vi "In_S1F2.vi"(8 "error in (no error)":errorcluster, 11 "S1 Message Class in":refnum<class "S1 Message Class.lvclass">) -> (0 "error out":errorcluster, 1 "OK?":bool, 2 "S1F2":T1, 3 "S1 Message Class out":refnum<class "S1 Message Class.lvclass">)   [LabVIEW 2020, in "SECS Communication.lvlib" / "S1 Message Class.lvclass"]
uses:
  S1 Message Class.lvclass
  D:/Dropbox/SECS/SECS_GEM v1.0.6/Com/SECS Communication/SECS-II Class/SECS-II Class.lvclass
  S1F2.ctl
  SECS-II Class/SECS-II Class.lvclass/SECS-II Class.ctl
  SECS-II Class/Variant To Data_ASCII.vi
  SECS-II Class/SECS-II Class.lvclass
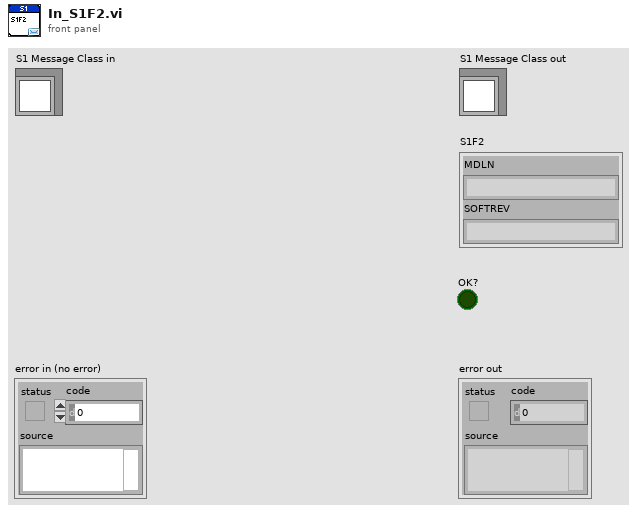
[diagram p1: front panel]
types:
  T1 = typedef "SECS Communication.lvlib/S1 Message Class.lvclass/S1F2.ctl" = cluster{"MDLN":string, "SOFTREV":string}
  T2 = typedef "SECS Communication.lvlib/SECS-II Class.lvclass/Message Data.ctl" = cluster{"Index":i32, "Data Item Format":T3, "Format Code":T4, "Parent Index":i32, "Child Index":i32[], "Data":variant}
  T3 = typedef "SECS Communication.lvlib/SECS-II Class.lvclass/Data Item Format.ctl" = enum16{"Data Type", "Value"}
  T4 = typedef "SECS Communication.lvlib/SECS-II Class.lvclass/Format Code.ctl" = enum16{"L", "A", "B", "Boolean", "J", "I1", "I2", "I4", "I8", "U1", "U2", "U4", "U8", "F4", "F8", "Char"}
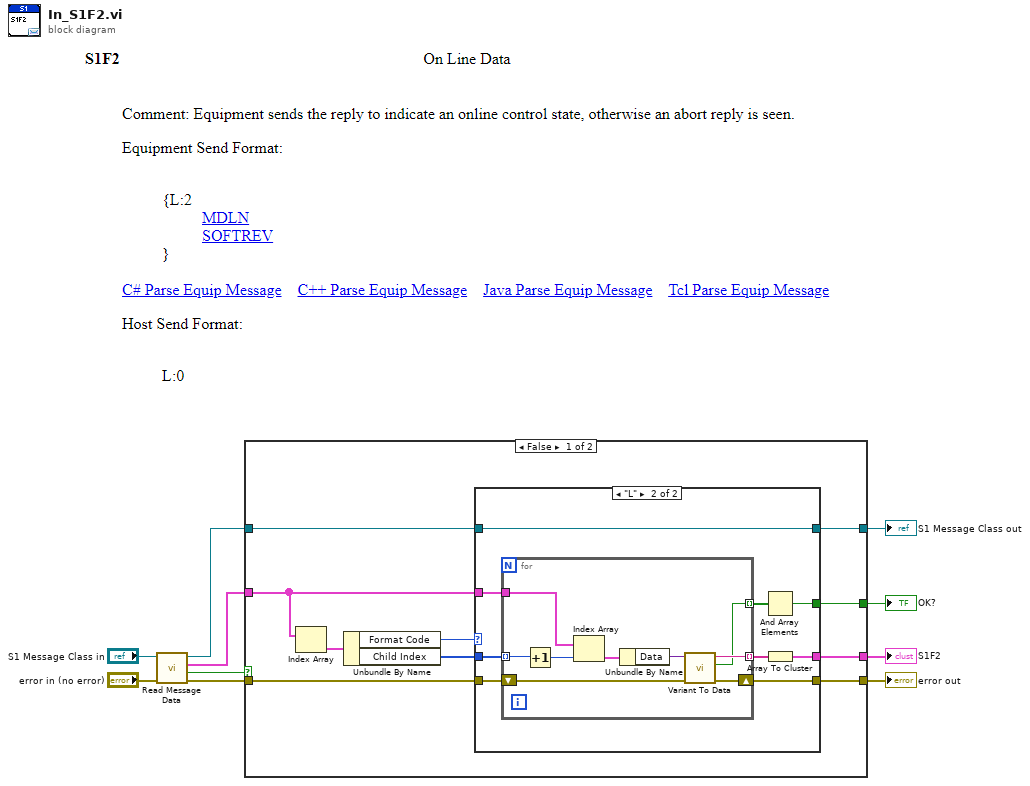
[diagram p0: block diagram]
diagram:
  n1 = call "Read Message Data.vi"("error in (no error)"="error in (no error)", "SECS-II Class in"="S1 Message Class in") -> ("error out"=w10:errorcluster, "Empty?"=w3:bool, "Message Data"=w4:T2[], "SECS-II Class out"=w7:refnum<class "S1 Message Class.lvclass">)  [unwired: 6 in]
  n2 = case shown="False" w3 {
    tunnel: w10 -> [w18 w42]
    tunnel: [w17 w42] -> w9
    tunnel: [w16 _] -> w8
    tunnel: w7 -> [w14 w41]
    tunnel: [w13 w41] -> w6
    tunnel: [w12 _] -> w5
    tunnel: w4 -> [w11 _]
    frame False {
      n3 = Index Array(array=w11) -> (element=w20:T2)  [unwired: 1 in]
      n4 = Unbundle By Name(w20) -> ("Format Code"=w15:T4, "Child Index"=w19:i32[])
      n5 = case shown="\"L\"" w15 {
        tunnel: w19 -> [_ w31]
        tunnel: w11 -> [_ w30]
        tunnel: w18 -> [w21 w29]
        tunnel: [w21 w28] -> w17
        tunnel: [_ w26] -> w16
        tunnel: w14 -> [w22 w25]
        tunnel: [w22 w25] -> w13
        tunnel: [_ w23] -> w12
        frame Default {
        }
        frame "L" {
          n6 = for {
            tunnel: w31 -> [w39] mode=indexing
            tunnel: w30 -> [w40]
            shift-right: [w34] -> w28
            shift-left: w29 -> [w36]
            tunnel: [w33] -> w27 mode=indexing
            tunnel: [w32] -> w24 mode=indexing
            n7 = Increment(x=w39) -> (x+1=w38:i32)
            n8 = Index Array(array=w40, index=w38) -> (element=w37:T2)
            n9 = Unbundle By Name(w37) -> ("Data"=w35:variant)
            n10 = call-poly "Variant To Data.vi"("error in (no error)"=w36, "Variant"=w35) -> ("error out"=w34:errorcluster, "OK?"=w32:bool, "Data"=w33:string)  [unwired: 7 in]
          }
          n11 = And Array Elements(Boolean array=w24) -> (logical AND=w23:bool)
          n12 = Array To Cluster(array=w27) -> (cluster=w26:cluster{"[0]":string, "[1]":string})
        }
      }
    }
    frame True {
    }
  }
  "error out" <- w9
  "S1 Message Class out" <- w6
  "S1F2" <- w8
  "OK?" <- w5
